vi "Configure Gyro.vi"(7 "Initialize":bool, 10 "data":dbl[](array[numeric]) format="%0.2f", 11 "Sensitivity (mV/°/s)":dbl=0.3) -> (3 "Rate of turn (°/s)":dbl)   [LabVIEW 2014]
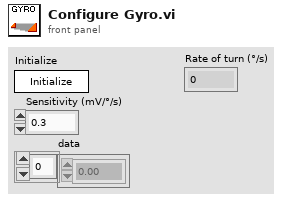
[diagram p1: front panel]
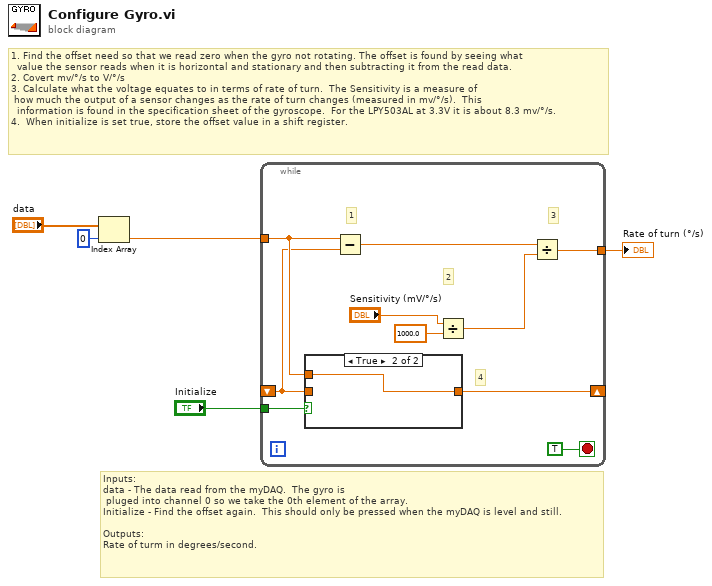
[diagram p0: block diagram]
diagram:
  # "Inputs:\ndata - The data read from the myDAQ.  The gyro is\n pluged into channel 0 so we take the 0th element of the array.\nInitialize - Find the offset again.  This should only be pressed when the myDAQ is level and still.\n\nOutputs:\nRate of turm in degrees/second."
  # "1.\tFind the offset need so that we read zero when the gyro not rotating. The offset is found by seeing what \n  value the sensor reads when it is horizontal and stationary and then subtracting it from the read data.\n2.\tCovert mv/°/s to V/°/s\n3.\tCalculate what the voltage equates to in terms of rate of turn.  The Sensitivity is a measure of\n how much the output of a sensor changes as the rate of turn changes (measured in mv/°/s).  This \n  information is found in the specification sheet of the gyroscope.  For the LPY503AL at 3.3V it is about 8.3 mv/°/s.\n4.\t When initialize is set true, store the offset value in a shift register."
  n1 = Index Array(array="data", index=0) -> (element=w1:dbl)
  n2 = while {
    tunnel: w1 -> [w8]
    tunnel: [w15] -> w5
    tunnel: "Initialize" -> [w9]
    shift-right: [w7] -> _
    shift-left: _ -> [w6]
    stop <- TRUE stop-if-true
    # "4"
    # "3"
    # "2"
    # "1"
    n3 = case shown="True" w9 {
      tunnel: w8 -> [_ w17]
      tunnel: [w16 w17] -> w7
      tunnel: w6 -> [w16 _]
      frame False {
      }
      frame True {
      }
    }
    n4 = Subtract(x=w8, y=w6) -> (x-y=w14:dbl)
    n5 = Divide(x="Sensitivity (mV/°/s)", y=1000.0) -> (x/y=w12:dbl)
    n6 = Divide(x=w14, y=w12) -> (x/y=w15:dbl)
  }
  "Rate of turn (°/s)" <- w5
